vi "Talk_to_ADAM_Module.vi"() -> ()   [LabVIEW 2010]
panel:
  in  "Command to send":string
  out "Comment out":string
  out "Reply":string
  in  "Port Name":string="MainNetwork"
  in  "Module Address":i32
  out "String to Write":string
  # "Happy reply starts \"!\"\nUnhappy reply starts \"?\""
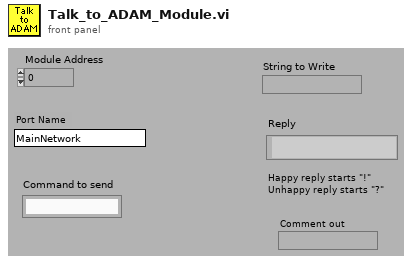
[diagram p1: front panel]
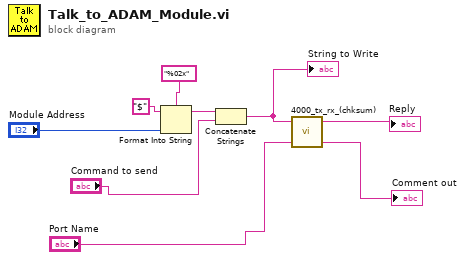
[diagram p0: block diagram]
diagram:
  n1 = Format Into String(format string="%02x", initial string="$", "Module Address") -> (resulting string=w3:string)  [unwired: 1 in, 1 out]
  n2 = Concatenate Strings(w3, "Command to send") -> (w1:string)
  "String to Write" <- w1
  n3 = call "4000_tx_rx_(chksum).vi"("Port Name"="Port Name", "Write String"=w1) -> ("Comment out"=→"Comment out":string, "Read"=→"Reply":string)  [unwired: 1 in, 1 out]
